vi "Save to File.vi"(10 "Text in":string="Test123", 11 "file path (use dialog)":path=path "C:/PotVals.txt") -> ()   [LabVIEW 2012]
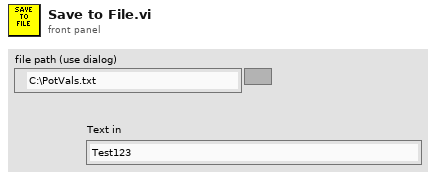
[diagram p1: front panel]
types:
  T1 = enum16{"open", "replace", "create", "open or create", "replace or create", "replace or create with confirmation"}
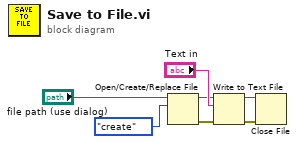
[diagram p0: block diagram]
diagram:
  n1 = Open/Create/Replace File(file path (use dialog)="file path (use dialog)", operation (0:open)=T1."create") -> (refnum out=w6:refnum<file>, error out=w5:errorcluster)  [unwired: 4 in, 1 out]
  n2 = Write to Text File(file (use dialog)=w6, text="Text in", error in=w5) -> (refnum out=w3:refnum<file>, error out=w4:errorcluster)  [unwired: 1 in, 1 out]
  n3 = Close File(refnum=w3, error in=w4) -> ()  [unwired: 2 out]
